vi "CT_SaveWaveformParams.vi"(8 "error in (no error)":errorcluster, 10 "Agilent Scintillator Scope Graph":waveform(dbl)[](graph)=[{"t0"=timestamp(-9.999999999998899e-05 s since 1904-01-01), "dt"=2e-09, "Y"=array[1000000 elements]}, {"t0"=timestamp(-9.999999999998899e-05 s since 1904-01-01), "dt"=2e-09, "Y"=array[1000000 elements]}], 11 "file path (dialog if empty)":path) -> (0 "error out":errorcluster)   [LabVIEW 2020]
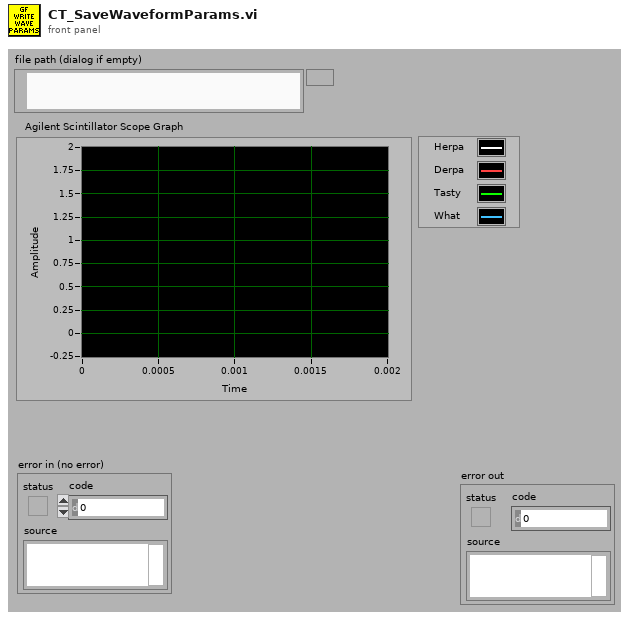
[diagram p1: front panel]
types:
  T1 = enum16{"open", "replace", "create", "open or create", "replace or create", "replace or create with confirmation"}
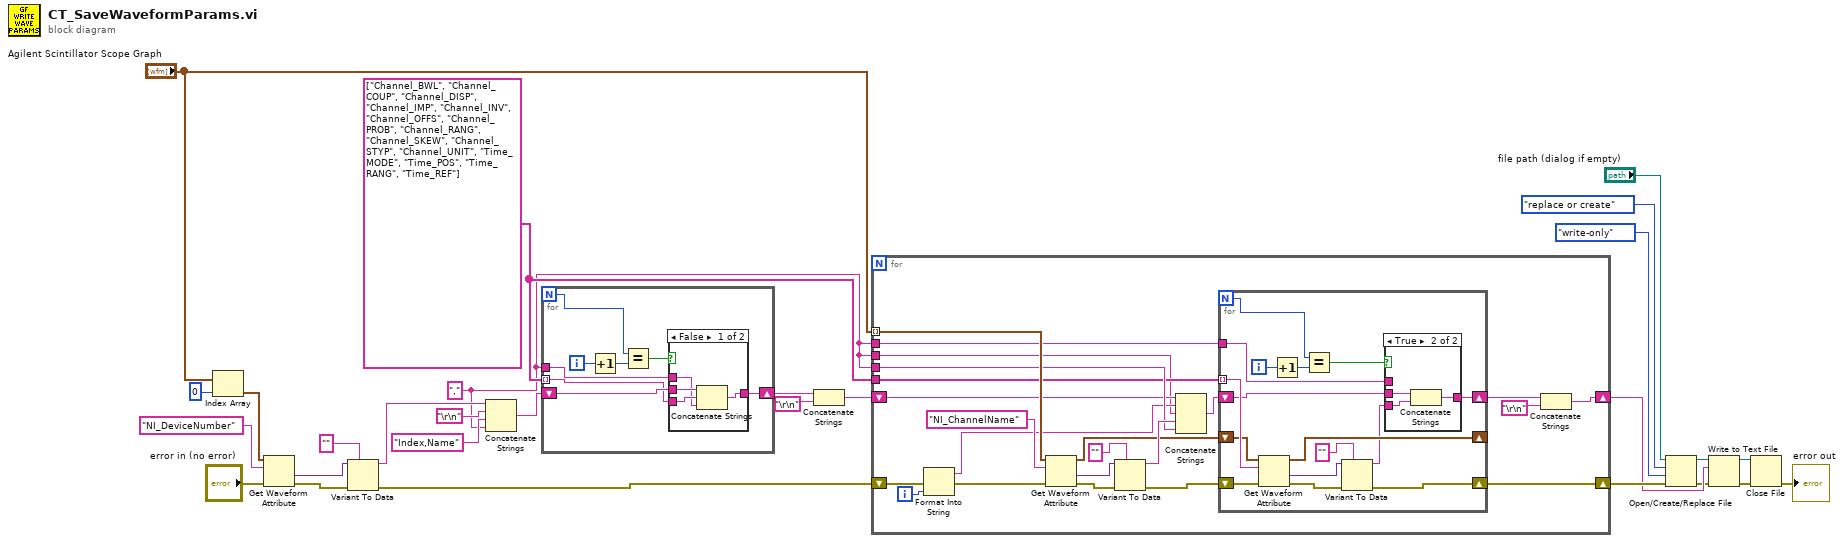
[diagram p0: block diagram]
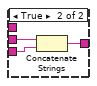
[diagram p2: hidden frame]
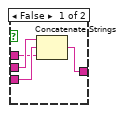
[diagram p3: hidden frame]
diagram:
  w1 = "," ("string")
  w8 = string[] ["Channel_BWL", "Channel_COUP", "Channel_DISP", "Channel_IMP", "Channel_INV", "Channel_OFFS", "Channel_PROB", "Channel_RANG", "Channel_SKEW", "Channel_STYP", "Channel_UNIT", "Time_MODE", "Time_POS", "Time_RANG", "Time_REF"]
  n1 = Index Array(array="Agilent Scintillator Scope Graph", index=0) -> (element=w6:waveform(dbl))
  n2 = Get Waveform Attribute(4:"error in (no error)", 6:"NI_DeviceNumber" ("name"), 7:w6) -> (0:w4:errorcluster, 1:w16:variant)  [unwired: 1 in, 2 out]
  n3 = Variant To Data(error in=w4, type="", Variant=w16) -> (data=w15:string, error out=w2:errorcluster)
  n4 = Concatenate Strings(w15, "\r\n", "Index,Name" ("string"), w1) -> (w13:string)
  n5 = for {
    N -> [w31]
    tunnel: w8 -> [w34] mode=indexing
    shift-right: [w36] -> w11
    shift-left: w13 -> [w35]
    tunnel: w1 -> [w33]
    i -> [w30]
    n6 = Increment(x=w30) -> (x+1=w32:i32)
    n7 = Equal?(x=w31, y=w32) -> (x = y?=w29:bool)
    n8 = case shown="False" w29 {
      tunnel: [w40 w43] -> w36
      tunnel: w35 -> [w39 w42]
      tunnel: w34 -> [w38 w41]
      tunnel: w33 -> [w37 _]
      frame False {
        n9 = Concatenate Strings(w39, w38, w37) -> (w40:string)
      }
      frame True {
        n10 = Concatenate Strings(w42, w41) -> (w43:string)
      }
    }
  }
  n11 = Concatenate Strings(w11, "\r\n") -> (w9:string)
  n12 = for {
    tunnel: "Agilent Scintillator Scope Graph" -> [w62] mode=indexing
    shift-right: [w50] -> w27
    shift-left: w2 -> [w48]
    shift-right: [w57] -> w25
    shift-left: w9 -> [w46]
    tunnel: w8 -> [w59]
    tunnel: w1 -> [w60]
    tunnel: w1 -> [w54]
    tunnel: w1 -> [w44]
    i -> [w49]
    n13 = Format Into String(error in=w48, w49) -> (resulting string=w45:string, error out=w47:errorcluster)  [unwired: 2 in]
    n14 = Get Waveform Attribute(4:w47, 6:"NI_ChannelName" ("name"), 7:w62) -> (0:w52:errorcluster, 1:w64:variant, 3:w58:waveform(dbl))  [unwired: 1 in, 1 out]
    n15 = Variant To Data(error in=w52, type="", Variant=w64) -> (data=w61:string, error out=w51:errorcluster)
    n16 = Concatenate Strings(w46, w45, w44, w61, w60) -> (w55:string)
    n17 = for {
      N -> [w73]
      tunnel: w59 -> [w79] mode=indexing
      shift-right: [w77] -> _
      shift-left: w58 -> [w78]
      tunnel: w54 -> [w66]
      shift-right: [w69] -> w53
      shift-left: w55 -> [w68]
      shift-right: [w74] -> w50
      shift-left: w51 -> [w76]
      i -> [w71]
      n18 = Get Waveform Attribute(4:w76, 6:w79, 7:w78) -> (0:w75:errorcluster, 1:w81:variant, 3:w77:waveform(dbl))  [unwired: 1 in, 1 out]
      n19 = Increment(x=w71) -> (x+1=w72:i32)
      n20 = Equal?(x=w73, y=w72) -> (x = y?=w70:bool)
      n21 = Variant To Data(error in=w75, type="", Variant=w81) -> (data=w67:string, error out=w74:errorcluster)
      n22 = case shown="True" w70 {
        tunnel: [w85 w88] -> w69
        tunnel: w68 -> [w84 w86]
        tunnel: w67 -> [w83 w87]
        tunnel: w66 -> [w82 _]
        frame False {
          n23 = Concatenate Strings(w84, w83, w82) -> (w85:string)
        }
        frame True {
          n24 = Concatenate Strings(w86, w87) -> (w88:string)
        }
      }
    }
    n25 = Concatenate Strings(w53, "\r\n") -> (w57:string)
  }
  n26 = Open/Create/Replace File(file path (use dialog)="file path (dialog if empty)", error in=w27, operation (0:open)=T1."replace or create", access (0:read/write)=enum16{"read/write", "read-only", "write-only"}."write-only") -> (refnum out=w26:refnum<file>, error out=w24:errorcluster)  [unwired: 2 in, 1 out]
  n27 = Write to Text File(file (use dialog)=w26, text=w25, error in=w24) -> (refnum out=w23:refnum<file>, error out=w22:errorcluster)  [unwired: 1 in, 1 out]
  n28 = Close File(refnum=w23, error in=w22) -> (error out=→"error out":errorcluster)  [unwired: 1 out]
